vi "Save Parameters to EEPROM.vi"(8 "error in (no error)":errorcluster, 10 "parameters":u16(ring) items=["default", "user"], 11 "VGC in":refnum<class "PL Inficon VGC.lvclass">) -> (0 "error out":errorcluster, 3 "VGC out":refnum<class "PL Inficon VGC.lvclass">)   [LabVIEW 2015, in "PL Inficon VGC.lvclass"]
doc: "Saves parameters to EEPROM."
uses:
  PL Inficon VGC.lvclass
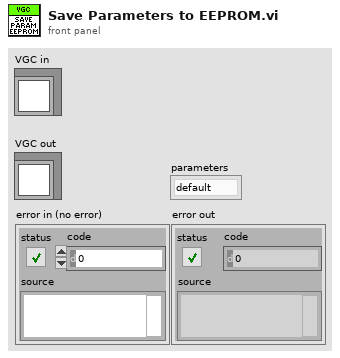
[diagram p1: front panel]
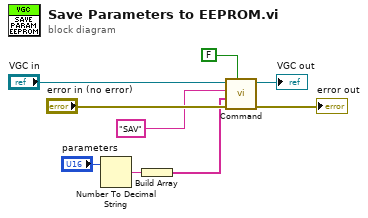
[diagram p0: block diagram]
diagram:
  n1 = Number To Decimal String(number="parameters") -> (decimal integer string=w5:string)  [unwired: 1 in]
  n2 = Build Array(w5) -> (w4:string[])
  n3 = call "Command.vi"("receive data (true)"=FALSE, "error in (no error)"="error in (no error)", "parameters"=w4, "command"="SAV", "VGC in"="VGC in") -> ("error out"=→"error out":errorcluster, "VGC out"=→"VGC out":refnum<class "PL Inficon VGC.lvclass">)  [unwired: 4 in, 1 out]
